vi "Apply Boolean Names.vi"(8 "error in":errorcluster, 9 "Enabled In":T1(array[ring]), 10 "Names in":string[](array[string]), 11 "Cluster_Refs in":refnum<vi>[](array[refnum])) -> (0 "error out":errorcluster, 1 "Enabled out":T1(array[ring]), 2 "Names out":string[](array[string]), 3 "Cluster_Refs Out":refnum<vi>[](array[refnum]))   [LabVIEW 2019, in "DIG_IO.lvlib" / "DIG_IO.lvclass"]
uses:
  Library/DIG_IO.lvclass
  Custom Controls/Single_Bank.ctl
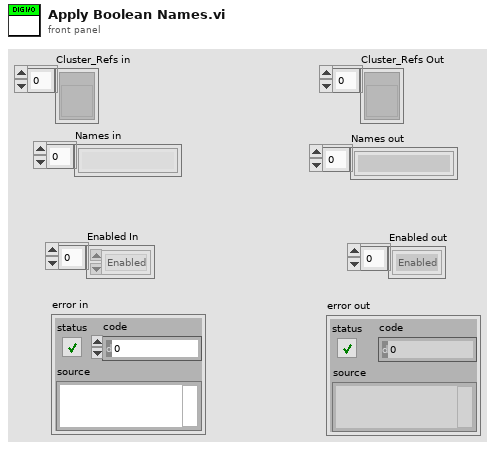
[diagram p1: front panel]
types:
  T1 = enum8{"Enabled", "Disabled", "Disabled and Grayed Out"}[]
  T2 = enum8{"Enabled", "Disabled", "Disabled and Grayed Out"}
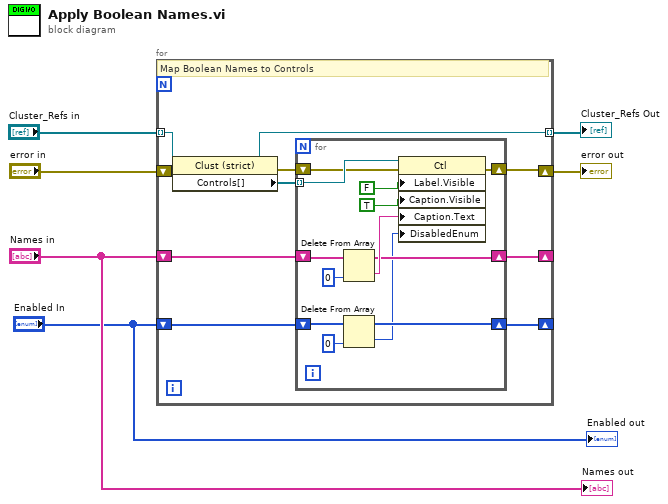
[diagram p0: block diagram]
diagram:
  n1 = for {
    shift-right: [w12] -> _
    shift-left: "Names in" -> [w13]
    tunnel: "Cluster_Refs in" -> [w16] mode=indexing
    tunnel: [w15] -> w4 mode=indexing
    shift-right: [w9] -> w2
    shift-left: "error in" -> [w11]
    shift-right: [w7] -> _
    shift-left: "Enabled In" -> [w8]
    # "Map Boolean Names to Controls"
    n2 = property class="Clust (strict)"(reference=w16, error in=w11) -> (reference out=w15:refnum<vi>, error out=w10:errorcluster, "Controls[]"=w14:refnum<vi>[])
    n3 = for {
      tunnel: w14 -> [w29] mode=indexing
      shift-right: [w23] -> w12
      shift-left: w13 -> [w26]
      shift-right: [w21] -> w9
      shift-left: w10 -> [w22]
      shift-right: [w18] -> w7
      shift-left: w8 -> [w20]
      n4 = Delete From Array(array=w26, index=0) -> (deleted portion=w24:string, array with subset deleted=w23:string[])  [unwired: 1 in]
      n5 = Delete From Array(array=w20, index=0) -> (deleted portion=w17:T2, array with subset deleted=w18:T1)  [unwired: 1 in]
      n6 = property class="Ctl"(reference=w29, error in=w22, "Label.Visible"=FALSE, "Caption.Visible"=TRUE, "Caption.Text"=w24, "DisabledEnum"=w17) -> (error out=w21:errorcluster)  [unwired: 1 out]
    }
  }
  "Cluster_Refs Out" <- w4
  "error out" <- w2
  "Names out" <- "Names in"
  "Enabled out" <- "Enabled In"
